vi "7.8- Convert neuron from Forebrain.vi"(0 "binary string":string) -> ()   [LabVIEW 2010]
uses:
  6-OCU Neurons/6.8-Forbrain to OCU neuron.ctl
  4-High Neurons/4.2-Where Sensor Typedef.ctl
  4-High Neurons/Current GPS Data.ctl
  3-Midbrain/3.2-Where/_typedefs/3.2.1-VectorNav Data.ctl
  6-OCU Neurons/6.3-Lidar Data.ctl
  6-OCU Neurons/6.3-What Reporting.ctl
  7.0-Global.vi
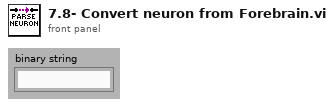
[diagram p1: front panel]
types:
  T1 = typedef "6.3-What Reporting.ctl" = cluster{"Local Map":dbl[][], "6.7-Lidar Data":T2}
  T2 = typedef "6.3-Lidar Data.ctl" = cluster{"Angle Array":dbl[], "Magnitude Array":dbl[]}
  T3 = typedef "6.8-Forbrain to OCU neuron.ctl" = cluster{"4.2-Where Am I? Sensor":T4, "6.7-Lidar Data":T2}
  T4 = typedef "4.2-Where Sensor Typedef.ctl" = cluster{"4.2.2- Current GPS Data":T5, "4.2.1-VectorNav Data":T6, "4.2.1-VectorNav Status":string}
  T5 = typedef "Current GPS Data.ctl" = cluster{"Lattitude (Decimal Degrees)":ext, "Longitude (Decimal Degrees)":ext, "EST Time":timestamp}
  T6 = typedef "3.2.1-VectorNav Data.ctl" = cluster{"Yaw":dbl, "Pitch":dbl, "Roll":dbl}
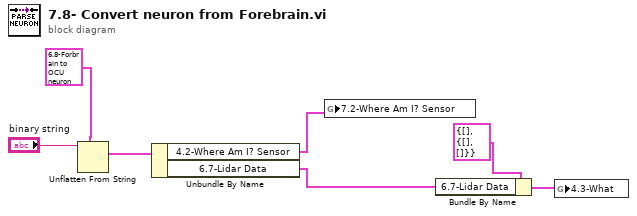
[diagram p0: block diagram]
diagram:
  n1 = Unflatten From String(type=T3 {"4.2-Where Am I? Sensor"={"4.2.2- Current GPS Data"={"Lattitude (Decimal Degrees)"=0.0, "Longitude (Decimal Degrees)"=0.0, "EST Time"=timestamp(0 s since 1904-01-01)}, "4.2.1-VectorNav Data"={"Yaw"=0.0, "Pitch"=0.0, "Roll"=0.0}, "4.2.1-VectorNav Status"=""}, "6.7-Lidar Data"={"Angle Array"=[], "Magnitude Array"=[]}} ("6.7-Forebrain to OCU Neuron"), binary string="binary string") -> (value=w5:T3)  [unwired: 3 in, 2 out]
  n2 = Unbundle By Name(w5) -> ("4.2-Where Am I? Sensor"=w1:T4, "6.7-Lidar Data"=w2:T2)
  n3 = global write "7.0-Global.vi" "7.2-Where Am I? Sensor"(w1) -> ()
  n4 = Bundle By Name(cluster=T1 {"Local Map"=[], "6.7-Lidar Data"={"Angle Array"=[], "Magnitude Array"=[]}} ("4.3-What"), "6.7-Lidar Data"=w2) -> (w3:T1)
  n5 = global write "7.0-Global.vi" "4.3-What"(w3) -> ()
